vi "resource array size.vi"(10 "Resources in":refnum<k20>[](array[refnum])) -> (2 "size":u32)   [LabVIEW 2015]
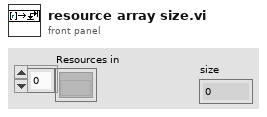
[diagram p1: front panel]
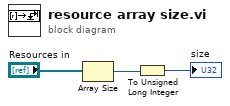
[diagram p0: block diagram]
diagram:
  n1 = Array Size(array="Resources in") -> (size(s)=w3:i32)
  n2 = To Unsigned Long Integer(number=w3) -> (unsigned 32bit integer=→"size":u32)
